vi "OAT Convert to Even Angle Signal (1 Channel).vi"(0 "scaled signal [EU]":waveform(dbl)={"t0"=timestamp(0 s since 1904-01-01), "dt"=0.0, "Y"=[]}, 1 "analysis method":u16(ring) items=["fast", "accurate"], 2 "reset? (F)":bool, 5 "speed profile":T6 {"speed [RPM]" format="%.2f"; "time [s]" format="%.2f"}, 7 "pulse/revolution (1)":i32=1, 11 "error in (no error)":errorcluster, 12 "max order (auto)":dbl, 13 "zero delay? (F)":bool) -> (4 "even-angle signal":cluster{"r0":dbl, "dr":dbl, "Y":dbl[]}={"r0"=0.0, "dr"=1.0, "Y"=[]} {"r0" format="%.2p"; "dr" format="%.2p"; "Y" format="%.2f"}, 6 "even-angle channel info":T2={"channel name"="", "description"="", " channel info"={"sensor sensitivity"=1000.0, "engineering units"=1, "dB reference"=1.0, "custom label"="EU", "weighting filter"=0, "pregain"=0.0}} {"channel info"."pregain" format="%.2f"; "channel info"."weighting filter" items=["Linear", "A-weighting", "B-weighting", "C-weighting", "ITU-R 468-4", "Dolby", "CCITT", "C-message", "Wb", "Wc", "Wd", "We", "Wf", "Wh", "Wj", "Wk", "Wm", "AES17 20 kHz lowpass", "AES17 40 kHz lowpass", "AES17 20 kHz highpass", "AES17 40 kHz highpass"]; "channel info"."dB reference" format="%^.1e"; "channel info"."engineering units" items=["custom..."=0, "V"=1, "A"=21, "C"=30, "pC"=31, "s"=32, "-"=29, "Pa"=2, "N"=20, "g"=3, "m/s^2"=4, "m/s"=5, "m"=6, "mm/s"=12, "mm"=13, "micron/s"=14, "micron"=15, "in/s^2"=7, "in/s"=8, "in"=9, "mil/s"=10, "mil"=11, "rad/s^2"=16, "rad/s"=17, "rad"=18, "deg/s^2"=26, "deg/s"=27, "deg"=28, "RPM"=22, "cycle/s^2"=23, "Hz"=24, "cycle"=25, "strain"=19]; "channel info"."sensor sensitivity" format="%#_5f"}, 8 "even-angle position info":T1, 14 "actual max order":dbl, 15 "error out":errorcluster)   [LabVIEW 2017, in "SoundVib_OrderTracking.lvlib"]
doc: "Converts an even-time-spaced scaled signal to an even-angle-spaced signal by resampling the acquired signal. Wire data to the <B>scaled signal [EU]</B> input to determine the polymorphic instance to use or manually select the instance."
uses:
  <vilib>/addons/Sound and Vibration/Order Analysis/Resample Order Tracking/SoundVib_OrderTracking.lvlib
  <vilib>/addons/Sound and Vibration/Order Analysis/Tach Process/SubVIs/speed profile.ctl
  <vilib>/addons/_NISVFA/_Shared subVIs/Controls/svc_Resampled Channel Info.ctl
  <vilib>/addons/_NISVFA/_Shared subVIs/Controls/svc_Channel Info.ctl
  <vilib>/addons/_NISVFA/_Shared subVIs/Controls/svc_Engineering Units Text Ring.ctl
  <vilib>/addons/_NISVFA/_Shared subVIs/Controls/svc_Weighting Filter Text Ring.ctl
  <vilib>/addons/Sound and Vibration/Order Analysis/Misc/OAT Position Info.ctl
  <vilib>/addons/_NISVFA/_Shared subVIs/Common/svc_Check for Waveform Parameter Continuity (no state).vi
  <vilib>/addons/Sound and Vibration/Order Analysis/Adv Resampling/oa_Adjust Resample State Info.vi
  <vilib>/addons/Sound and Vibration/Order Analysis/Misc/OAT Error Information.vi
  <vilib>/addons/Sound and Vibration/Order Analysis/Adv Resampling/OAT Prepare Resample Data.vi
  <vilib>/addons/_NISVFA/_Shared subVIs/Common/svc_Engineering Units to Unit Label.vi
  <vilib>/addons/_NISVFA/_Shared subVIs/Common/svc_Unit Label to Engineering Units.vi
  <vilib>/addons/Sound and Vibration/Order Analysis/Resample Order Tracking/SoundVib_Resampling.lvlib
  <vilib>/addons/Sound and Vibration/Order Analysis/Tach Process/SoundVib_TachProcess.lvlib
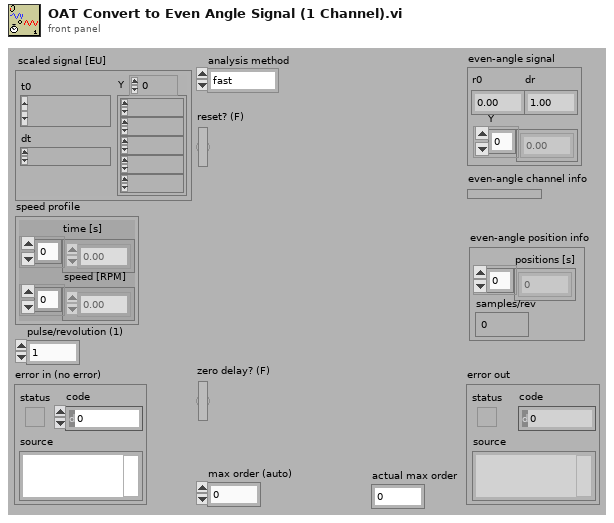
[diagram p1: front panel]
types:
  T1 = typedef "OAT Position Info.ctl" = cluster{"positions [s]":dbl[], "samples/rev":dbl}
  T2 = typedef "svc_Resampled Channel Info.ctl" = cluster{"channel name":string, "description":string, " channel info":T3}
  T3 = typedef "svc_Channel Info.ctl" = cluster{"sensor sensitivity":dbl, "engineering units":T4, "dB reference":dbl, "custom label":string, "weighting filter":T5, "pregain":dbl}
  T4 = typedef "svc_Engineering Units Text Ring.ctl" = u16
  T5 = typedef "svc_Weighting Filter Text Ring.ctl" = u16
  T6 = typedef "SoundVib_TachProcess.lvlib/speed profile.ctl" = cluster{"time [s]":dbl[], "speed [RPM]":dbl[]}
  T7 = cluster{"dt":bool, "t0 continuity":bool, "array length":bool, "channel info":bool, "name":bool}
  T8 = typedef "OAT Resample Filter Prototype.ctl" = cluster{"left wing":dbl[], "increment":dbl[], "max dec":i32, "timing jitter":enum32{"Interpolation", "Rounding"}, "band limiting?":bool}
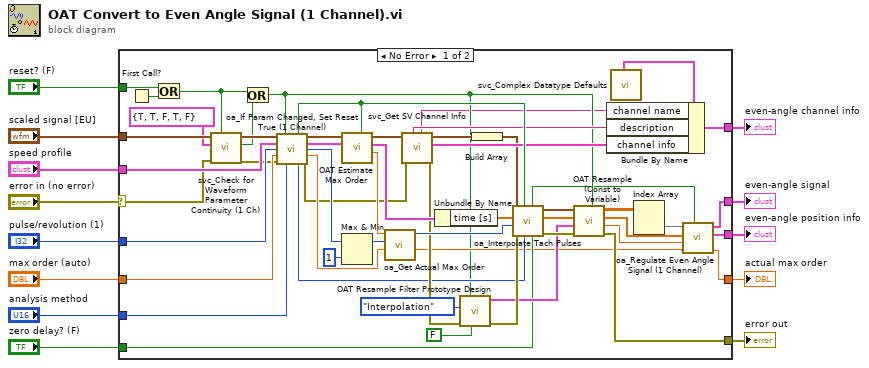
[diagram p0: block diagram]
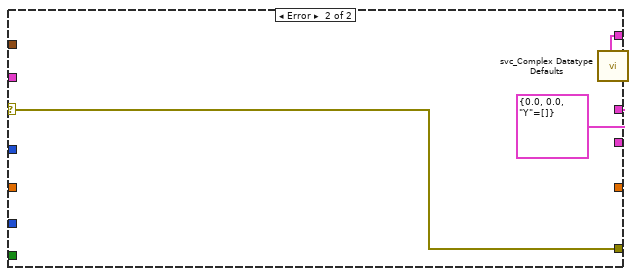
[diagram p2: hidden frame]
diagram:
  n1 = case shown="No Error" "error in (no error)" {
    selector: "error in (no error)" -> [w26 w69]
    tunnel: "pulse/revolution (1)" -> [w50 _]
    tunnel: "max order (auto)" -> [w48 _]
    tunnel: [w20 cluster{dbl, dbl, "Y":dbl[]} {0.0, 0.0, "Y"=[]}] -> w11
    tunnel: "scaled signal [EU]" -> [w30 _]
    tunnel: "speed profile" -> [w45 _]
    tunnel: [w64 w69] -> w8
    tunnel: "analysis method" -> [w41 _]
    tunnel: [w54 w68] -> w5
    tunnel: [w19 _] -> w4
    tunnel: [w18 _] -> w3
    tunnel: "reset? (F)" -> [w46 _]
    tunnel: "zero delay? (F)" -> [w31 _]
    frame No Error {
      n2 = First Call?() -> (First Call?: T/F=w53:bool)
      n3 = Or(x=w46, y=w53) -> (x .or. y?=w28:bool)
      n4 = call <vilib>:"svc_Check for Waveform Parameter Continuity (1 Ch).vi"("restart averaging (F)"=w28, "error in (no error)"=w26, "checks for channel parameter change"=T7 {"dt"=TRUE, "t0 continuity"=TRUE, "array length"=FALSE, "channel info"=TRUE, "name"=FALSE}, "scaled signal [EU]"=w30) -> ("error out"=w25:errorcluster, "waveform parameter changed"=w27:bool, "dup scaled signal [EU]"=w29:waveform(dbl))  [unwired: 2 in, 3 out]
      n5 = Or(x=w28, y=w27) -> (x .or. y?=w17:bool)
      n6 = call <vilib>:"oa_If Param Changed, Set Reset True (1 Channel).vi"("scaled signal in [EU]"=w29, "reset in"=w17, "speed profile"=w45, "pulse/revolution in (1)"=w50, "max order in (auto)"=w48, "error in (no error)"=w25, "analysis method in"=w41) -> ("reset out"=w52:bool, "scaled signal out [EU]"=w51:waveform(dbl), "speed profile out"=w44:T6, "pulse/revolution out (1)"=w49:i32, "max order out (auto)"=w47:dbl, "analysis method out"=w40:u16, "error out"=w39:errorcluster)  [unwired: 2 in]
      n7 = call <vilib>:"OAT Estimate Max Order.vi"("reset? (True)"=w52, "speed profile in"=w44, "scaled signal [EU] in"=w51) -> ("max suggested order"=w65:dbl, "speed profile out"=w66:T6, "scaled signal [EU] out"=w56:waveform(dbl))  [unwired: 5 in, 1 out]
      n8 = Max & Min(x=w49, y=1) -> (max(x,y)=w57:i32)  [unwired: 1 out]
      n9 = call <vilib>:"oa_Get Actual Max Order.vi"("max order (auto)"=w47, "pulse/revolution (1)"=w57, "max suggested order"=w65) -> ("new pulse/revolution"=w21:dbl, "interpolation factor"=w58:i32)  [unwired: 7 in]
      n10 = call <vilib>:"svc_Get SV Channel Info.vi"("error in (no error)"=w39, "scaled signal [EU]"=w56) -> ("error out"=w42:errorcluster, "channel info"=w37:T3, "dup scaled signal [EU]"=w55:waveform(dbl), "channel name"=w15:string, "channel description"=w36:string)  [unwired: 4 in, 1 out]
      n11 = Unbundle By Name(w66) -> ("time [s]"=w33:dbl[])
      n12 = call <vilib>:"OAT Resample Filter Prototype Design.vi"("alias free"=FALSE ("alias protect in final transition"), "reset? (True)"=w17, "error in (no error)"=w42, "timing jitter"=enum32{"Interpolation", "Rounding"}."Interpolation") -> ("error out"=w63:errorcluster, "filter prototype"=w60:T8)  [unwired: 5 in, 1 out]
      n13 = Build Array(w55) -> (w35:waveform(dbl)[])
      n14 = call <vilib>:"oa_Interpolate Tach Pulses.vi"("zero delay? (F)"=w31, "resolution"=w40, "reset? (True)"=w52, "error in (no error)"=w63, "interpolation factor"=w58, "pulse positions [s]"=w33, "scaled signals (EU)"=w35) -> ("error out"=w62:errorcluster, "interpolated pulse positions[s]"=w32:dbl[], "dup scaled signals (EU)"=w34:waveform(dbl)[], "reset out"=w16:bool)  [unwired: 1 in]
      n15 = call <vilib>:"OAT Resample (Const to Variable).vi"("reset? (True)"=w17, "error in (no error)"=w62, "filter prototype"=w60, "time"=w32, "scaled signals (EU)"=w34) -> ("error out"=w64:errorcluster, "offset"=w22:dbl, "time stamps"=w23:dbl[], "Y"=w59:dbl[][])  [unwired: 3 in]
      n16 = call <vilib>:"svc_Complex Datatype Defaults.vi"() -> ("resampled channel info"=w38:T2)  [unwired: 11 in, 8 out]
      n17 = Bundle By Name(cluster=w38, "channel name"=w15, "description"=w36, "channel info"=w37) -> (w54:T2)
      n18 = Index Array(array=w59) -> (element=w24:dbl[])  [unwired: 2 in]
      n19 = call <vilib>:"oa_Regulate Even Angle Signal (1 Channel).vi"("reset?"=w16, "samples/rev"=w21, "offset"=w22, "time stamps"=w23, "Data"=w24) -> ("actual max order"=w18:dbl, "even-angle position info"=w19:T1, "even-angle signal"=w20:cluster{"r0":dbl, "dr":dbl, "Y":dbl[]})  [unwired: 4 in]
    }
    frame Error {
      n20 = call <vilib>:"svc_Complex Datatype Defaults.vi"() -> ("resampled channel info"=w68:T2)  [unwired: 11 in, 8 out]
    }
  }
  "even-angle signal" <- w11
  "even-angle channel info" <- w5
  "even-angle position info" <- w4
  "error out" <- w8
  "actual max order" <- w3
